vi "SetObject_GObject.vi"(5 "GObject":refnum<class "GObject.lvclass">, 6 "error in":errorcluster, 9 "VI Interpreter in":refnum<class "VI Interpreter.lvclass">) -> (0 "error out":errorcluster, 3 "VI Interpreter out":refnum<class "VI Interpreter.lvclass">)   [LabVIEW 2014, in "VI Interpreter.lvclass"]
uses:
  VI Interpreter.lvclass
  GObject/GObject.lvclass
  VI Interpreter.lvclass/VI Interpreter.ctl
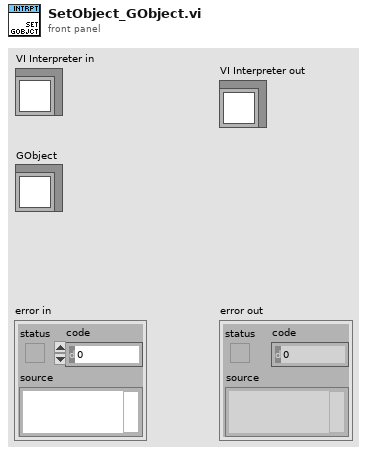
[diagram p1: front panel]
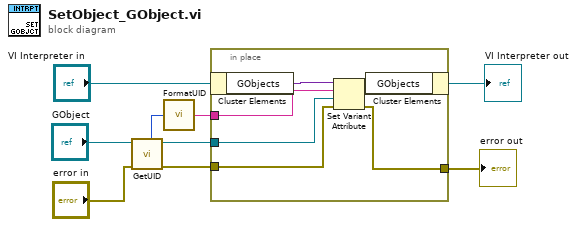
[diagram p0: block diagram]
diagram:
  n1 = call-dynamic "GetUID.vi"("error in"="error in", "GObject in"="GObject") -> ("error out"=w2:errorcluster, "GObject out"=w3:refnum<class "GObject.lvclass">, "UID"=w4:i32)  [unwired: 5 in]
  n2 = call "FormatUID.vi"("UID"=w4) -> ("Name"=w1:string)
  n3 = in-place {
    in-place-border: [w14] -> w7
    in-place-border: w2 -> [w12]
    in-place-border: w3 -> [w11]
    in-place-border: w1 -> [w10]
    n4 = in-place-cluster #1("VI Interpreter in") -> ("GObjects"=w15:variant)
    n5 = Set Variant Attribute(Variant=w15, name=w10, value=w11, error in=w12) -> (Variant out=w13:variant, error out=w14:errorcluster)  [unwired: 1 out]
    n6 = in-place-cluster #1("GObjects"=w13) -> (→"VI Interpreter out":refnum<class "VI Interpreter.lvclass">)
  }
  "error out" <- w7
